vi "DFD IIR Comb Design by f and BW.vi"(6 "fs [Hz]":dbl=1.0 format="%.2f", 7 "filter type":T1(ring), 8 "error in (no error)":errorcluster, 9 "Ab [dB]":dbl=3.010299956639812 format="%#.6g", 10 "Df [Hz]":dbl=0.02 format="%#_2f", 11 "f0 [Hz]":dbl=0.1 format="%.2f") -> (0 "error out":errorcluster, 3 "filter out":T2={"mSRate_Fs"=1.0, "mSRate_Version"="2.0", "mSRate_Comments"="", "mSRate_OrgCoef"={"type"=enum."Undefined", "gain"=1.0, "coef a (k)"=[], "coef b (v)"=[]}, "mSRate_CurCoef"={"type"=enum."Undefined", "gain"=1.0, "coef a (k)"=[], "coef b (v)"=[]}, "mSRate_Quantized?"=FALSE, "mSRate_QCoef"={"type"=enum."Undefined", "gain"=1.0, "coef a (k)"=[], "coef b (v)"=[]}, "mSRate_QSettings"=[], "mSRate_Order"=0, "mSRate_Scaling"={"mSRate_ScaleByPowerOf2?"=FALSE, "mSRate_ScaleType"=enum."No Norm"}} {"mSRate_QSettings"."source" items=["Coef a/k"=0, "Coef b/v"=7, "Input"=1, "Output"=2, "Multiplicand"=3, "Product"=4, "Sum"=5, "Delay"=6, "Gain"=8]})   [LabVIEW 2017, in "NI_DigFilterLicensed.lvlib"]
doc: "Creates an infinite impulse response (IIR) comb filter. You must manually select the polymorphic instance you want to use."
uses:
  <vilib>/addons/Digital Filter Design/NI_DigFilterLicensed.lvlib
  <vilib>/addons/Digital Filter Design/_Objects.llb/DFD Filter Obj.ctl
  <vilib>/addons/Digital Filter Design/_Objects.llb/DFD Filter Coef.ctl
  <vilib>/addons/Digital Filter Design/_Objects.llb/DFD Filter Structure Type Selector.ctl
  <vilib>/addons/Digital Filter Design/_Objects.llb/dfd_Internal Quantization Settings.ctl
  <vilib>/addons/Digital Filter Design/_Objects.llb/dfd_Internal Quantization Srcs.ctl
  <vilib>/addons/Digital Filter Design/_Objects.llb/DFD Coef Norm Type.ctl
  <vilib>/addons/Digital Filter Design/NI_DigFilter_Design.lvlib
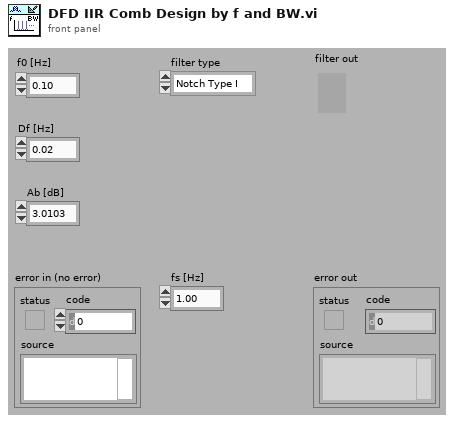
[diagram p1: front panel]
types:
  T1 = enum16{"Notch Type I", "Notch Type II", "Peak Type I", "Peak Type II"}
  T2 = typedef "NI_DigFilterLicensed.lvlib/DFD Filter Obj.ctl" = cluster{"mSRate_Fs":dbl, "mSRate_Version":string, "mSRate_Comments":string, "mSRate_OrgCoef":T3, "mSRate_CurCoef":T3, "mSRate_Quantized?":bool, "mSRate_QCoef":T3, "mSRate_QSettings":T5[], "mSRate_Order":i32, "mSRate_Scaling":cluster{"mSRate_ScaleByPowerOf2?":bool, "mSRate_ScaleType":T7}}
  T3 = typedef "NI_DigFilterLicensed.lvlib/DFD Filter Coef.ctl" = cluster{"type":T4, "gain":dbl, "coef a (k)":dbl[], "coef b (v)":dbl[]}
  T4 = typedef "NI_DigFilterLicensed.lvlib/DFD Filter Structure Type Selector.ctl" = enum16{"Undefined", "FIR Direct Form", "FIR Direct Form Transposed", "FIR Symmetric", "FIR Antisymmetric", "IIR Direct Form I", "IIR Direct Form I Transposed", "IIR Direct Form II", "IIR Direct Form II Transposed", "IIR Cascaded Second Order Sections Form I", "IIR Cascaded Second Order Sections Form I Transposed", "IIR Cascaded Second Order Sections Form II", "IIR Cascaded Second Order Sections Form II Transposed", "Lattice Allpass (basic sections)", "Lattice Allpass (one multiplier sections)", "Lattice Allpass (normalized sections)", "Lattice AR (basic sections)", "Lattice AR (one multiplier sections)", "Lattice AR (normalized sections)", "Lattice MA (minimum phase)", "Lattice MA (maximum phase)", "Lattice ARMA (basic sections)", "Lattice ARMA (one multiplier sections)", "Lattice ARMA (normalized sections)"}
  T5 = typedef "NI_DigFilterLicensed.lvlib/dfd_Internal Quantization Settings.ctl" = cluster{"source":T6, "wl":i16, "iwl":i16, "overflow mode":enum16{"Saturation", "Wrap"}, "rounding mode":enum16{"Nearest", "Truncation"}, "signed?":bool}
  T6 = typedef "NI_DigFilterLicensed.lvlib/dfd_Internal Quantization Srcs.ctl" = u16
  T7 = typedef "NI_DigFilterLicensed.lvlib/DFD Coef Norm Type.ctl" = enum16{"No Norm", "Time Domain 1-Norm", "Time Domain 2-Norm", "Time Domain Inf-Norm"}
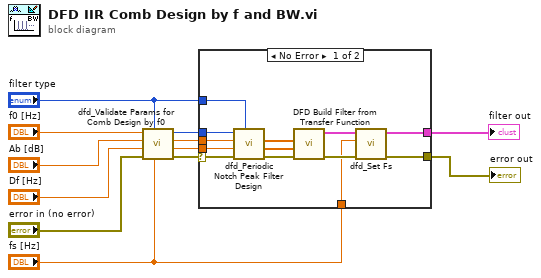
[diagram p0: block diagram]
diagram:
  n1 = call <vilib>:"dfd_Validate Params for Comb Design by f0.vi"("fs [Hz]"="fs [Hz]", "filter type"="filter type", "error in (no error)"="error in (no error)", "bandwidth [Hz]"="Df [Hz]", "Ab [dB]"="Ab [dB]", "f0 [Hz]"="f0 [Hz]") -> ("error out"=w1:errorcluster, "normalized BW [rad/s]"=w5:dbl, "dup Ab [dB]"=w6:dbl, "dup order"=w7:i32)  [unwired: 2 out]
  n2 = case shown="No Error" w1 {
    selector: w1 -> [w13 w25]
    tunnel: [w20 w25] -> w12
    tunnel: [w19 _] -> w11
    tunnel: "filter type" -> [w18 _]
    tunnel: w7 -> [w17 _]
    tunnel: w6 -> [w16 _]
    tunnel: w5 -> [w15 _]
    tunnel: "fs [Hz]" -> [w14 _]
    frame No Error {
      n3 = call <vilib>:"dfd_Periodic Notch Peak Filter Design.vi"("filter type"=w18, "normalized BW [rad/s]"=w15, "Ab [dB]"=w16, "order"=w17) -> ("denominator"=w23:dbl[], "numerator"=w24:dbl[])  [unwired: 2 in, 4 out]
      n4 = call <vilib>:"DFD Build Filter from Transfer Function.vi"("error in (no error)"=w13, "denominator"=w23, "numerator"=w24) -> ("error out"=w21:errorcluster, "filter out"=w22:T2)  [unwired: 1 in, 6 out]
      n5 = call <vilib>:"dfd_Set Fs.vi"("error in (no error)"=w21, "fs [Hz]"=w14, "filter in"=w22) -> ("error out"=w20:errorcluster, "filter out"=w19:T2)  [unwired: 7 out]
    }
    frame Error {
    }
  }
  "filter out" <- w11
  "error out" <- w12
